vi "nominal channel get.vi"(7 "out_channel":i32, 8 "error in (no error)":errorcluster, 9 "name":string, 10 "data_source_rid":string, 11 "client":i32) -> (0 "error out":errorcluster, 3 "function return":i32, 5 "out_channel out":i32)   [LabVIEW 2020, in "client.lvlib"]
doc: "int32_t nominal_channel_get(int32_t client,\n const char *data_source_rid,\n const char *name,\n int32_t *out_channel);"
uses:
  client.lvlib
  bin/nominalClient_64.dll
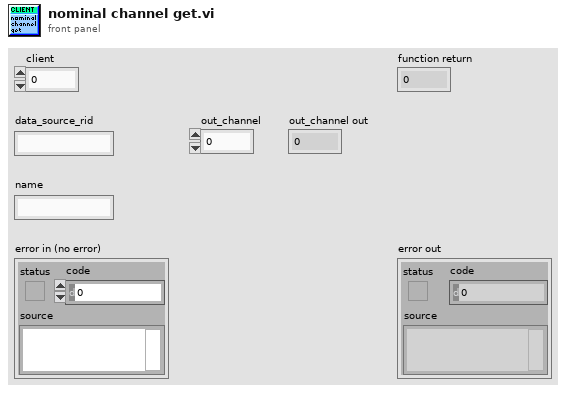
[diagram p1: front panel]
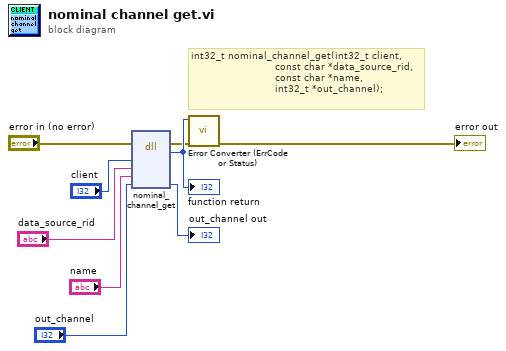
[diagram p0: block diagram]
diagram:
  # "int32_t nominal_channel_get(int32_t client,\n                            const char *data_source_rid,\n                            const char *name,\n                            int32_t *out_channel);"
  n1 = dll-call lib="C:/code/labview-client-rs/lv_src/bin/nominalClient_*.*" fn="nominal_channel_get"(error in="error in (no error)", "client"="client", "data_source_rid"="data_source_rid", "name"="name", "out_channel"="out_channel") -> (error out=w2:errorcluster, w9:i32, "out_channel"=→"out_channel out":i32)  [unwired: 5 in, 1 out]
  "function return" <- w9
  n2 = call "Error Converter (ErrCode or Status).vi"("error in (no error)"=w2, "error code"=w9) -> ("error out"=→"error out":errorcluster)  [unwired: 9 in]
